vi "Recall 6-Contact Sample Hall Results.vi"() -> (2 "6-Contact Sample Hall Results":T1)   [LabVIEW 2016, in "Hall Effect Library.lvlib"]
uses:
  Hall Effect Library.lvlib
  Private/Global Variables/Hall Effect Data.vi
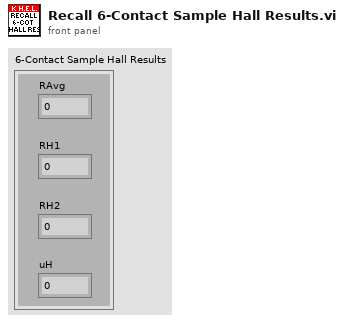
[diagram p1: front panel]
types:
  T1 = cluster{"RAvg":dbl, "RH1":dbl, "RH2":dbl, "uH":dbl}
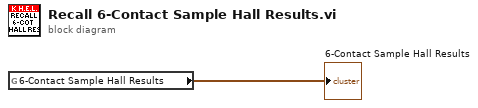
[diagram p0: block diagram]
diagram:
  n1 = global read "Hall Effect Data.vi" "6-Contact Sample Hall Results"() -> (→"6-Contact Sample Hall Results":T1)
